vi "Atto DRY Interface get Reservoir Tset Warm Magnet.vi"(8 "error in (no error)":errorcluster, 11 "ReservoirTsetWarmMagnetK":sgl) -> (0 "error out":errorcluster, 2 "function return":i32, 3 "ReservoirTsetWarmMagnetK out":sgl)   [LabVIEW 2016, in "attoDRYLib.lvlib"]
doc: "int32_t __cdecl AttoDRY_Interface_getReservoirTsetWarmMagnet(\n float *ReservoirTsetWarmMagnetK);"
uses:
  <userlib>/attoDRYLib/attoDRYLib.lvlib
  <userlib>/attoDRYLib/attoDRYLib.dll
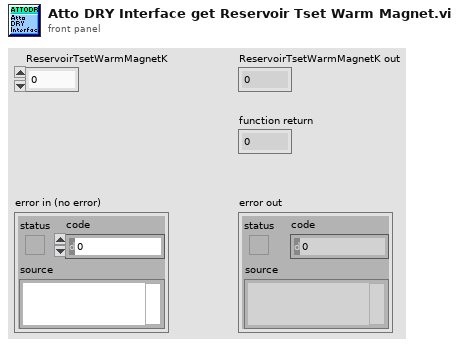
[diagram p1: front panel]
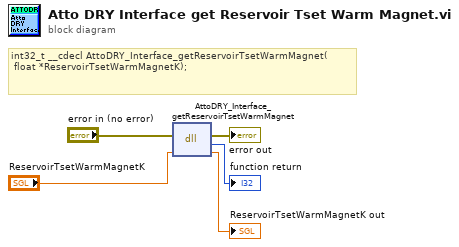
[diagram p0: block diagram]
diagram:
  # "int32_t __cdecl AttoDRY_Interface_getReservoirTsetWarmMagnet(\n\tfloat *ReservoirTsetWarmMagnetK);"
  n1 = dll-call lib="C:/Program Files (x86)/National Instruments/LabVIEW 2016/user.lib/attoDRYLib/attoDRYLib.*" fn="AttoDRY_Interface_getReservoirTsetWarmMagnet"(error in="error in (no error)", "ReservoirTsetWarmMagnetK"="ReservoirTsetWarmMagnetK") -> (error out=→"error out":errorcluster, →"function return":i32, "ReservoirTsetWarmMagnetK"=→"ReservoirTsetWarmMagnetK out":sgl)  [unwired: 2 in, 1 out]
